vi "rvc Blackbody.vi"() -> ()   [LabVIEW 2013]
uses:
  <vilib>/gmath/NumericalOptimization/Nonlinear Curve Fit LM formula string.vi
  <vilib>/gmath/NI_Gmath.lvlib
panel:
  out "I [W/cm/mm] fit":dbl[](array[numeric])=[1.6042937075355224e-42, 2.42119911255193e-16, 5.389391654786257e-08, 0.0005258099860789816, 0.10108074293224578, 2.8467891520795487, 27.40956542172593, 136.97870458059597, 446.5682313746935] format="%#.2e"
  in  "I [W/cm/mm]":dbl[](array[numeric])=[1.3e-11, 0.0054, 1.9, 32.0, 96.0, 220.0, 300.0, 340.0, 350.0] format="%.2e"
  in  "l [cm]":dbl[](array[numeric])=[1e-05, 2e-05, 3e-05, 4e-05, 5e-05, 6e-05, 7e-05, 8e-05, 9e-05] format="%#.2e"
  in  "Tolerance":dbl=0.01
  in  "Max iteration":i32=1000000
  out "par fit":dbl[](array[numeric])=[1128.5478560548609] caption="Best fit\nparameters"
  in  "par init":dbl[](array[numeric])=[3100.0] caption="Initial\nparameters"
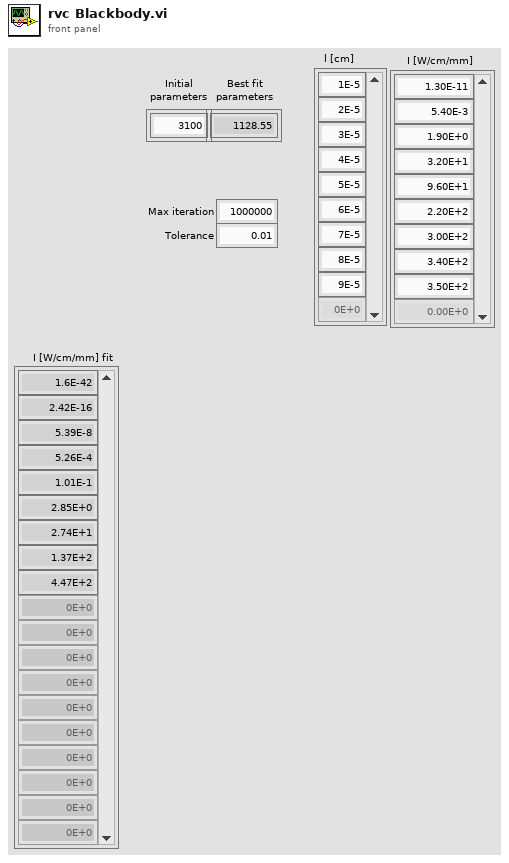
[diagram p1: front panel]
types:
  T1 = cluster{"model":string, "Parameters":string[], "x":string}
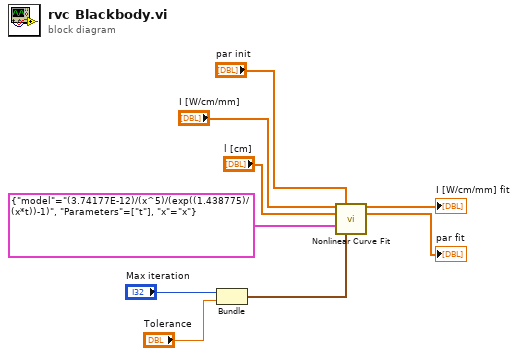
[diagram p0: block diagram]
diagram:
  n1 = Bundle("Max iteration"="Max iteration", "Tolerance"="Tolerance") -> (w2:cluster{"Max iteration":i32, "Tolerance":dbl})  [unwired: 1 in]
  n2 = call-poly <vilib>:"Nonlinear Curve Fit.vi"("Y"="I [W/cm/mm]", "initial parameters"="par init", "X"="l [cm]", "model description"=T1 {"model"="(3.74177E-12)/(x^5)/(exp((1.438775)/(x*t))-1)", "Parameters"=["t"], "x"="x"}, "termination"=w2) -> ("best nonlinear fit"=→"I [W/cm/mm] fit":dbl[], "best fit parameters"=→"par fit":dbl[])  [unwired: 6 in, 3 out]
